vi "MemBlockTagList(TimeStamps).vi"(7 "方法":enum16{"初始化", "获取索引"}(ring), 8 "error in (no error)":errorcluster caption="错误输入（无错误）", 10 "标签":string, 11 "内存块标签列表":T1(array[cluster])) -> (0 "error out":errorcluster caption="错误输出", 1 "标签索引":i32, 3 "默认值":timestamp[](array[timestamp]))   [LabVIEW 2013, in "MemBlock.lvlib"]
uses:
  MemBlock.lvlib
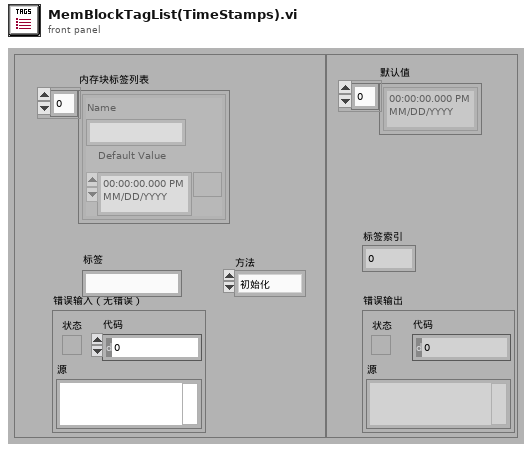
[diagram p1: front panel]
types:
  T1 = cluster{"Name":string, "Default Value":timestamp}[]
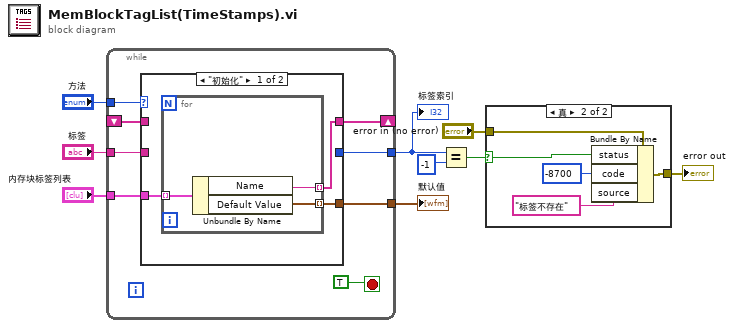
[diagram p0: block diagram]
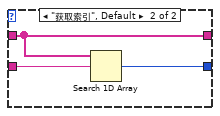
[diagram p3: hidden frame]
diagram:
  n1 = while {
    shift-right: [w13] -> _
    shift-left: _ -> [w15]
    tunnel: "方法" -> [w16]
    tunnel: "内存块标签列表" -> [w14]
    tunnel: [w12] -> w7
    tunnel: "标签" -> [w11]
    tunnel: [w10] -> w5
    stop <- TRUE stop-if-true
    n2 = case shown="\"初始化\"" w16 {
      tunnel: w15 -> [_ w24]
      tunnel: w14 -> [w20 _]
      tunnel: [w19 w24] -> w13
      tunnel: [w18 _] -> w12
      tunnel: w11 -> [_ w26]
      tunnel: [_ w25] -> w10
      frame "初始化" {
        n3 = for {
          tunnel: w20 -> [w23] mode=indexing
          tunnel: [w22] -> w19 mode=indexing
          tunnel: [w21] -> w18 mode=indexing
          n4 = Unbundle By Name(w23) -> ("Name"=w22:string, "Default Value"=w21:timestamp)
        }
      }
      frame "获取索引", Default {
        n5 = Search 1D Array(1D array=w24, element=w26) -> (index of element=w25:i32)  [unwired: 1 in]
      }
    }
  }
  "标签索引" <- w5
  "默认值" <- w7
  n6 = Equal?(x=w5, y=-1) -> (x = y?=w3:bool)
  n7 = case shown="真" w3 {
    selector: w3 -> [_ w32]
    tunnel: [w27 w31] -> w2
    tunnel: "error in (no error)" -> [w27 w28]
    frame False {
    }
    frame True {
      n8 = Bundle By Name(cluster=w28, "status"=w32, "code"=-8700, "source"="标签不存在") -> (w31:errorcluster)
    }
  }
  "error out" <- w2
